vi "Get Log File Name And Path.vi"(6 "timeout (ms)":i32=-1, 8 "error in (no error)":errorcluster, 11 "FlexLogger_gRPCAPI in":refnum<class "FlexLogger_gRPC.lvclass">) -> (0 "error out":errorcluster, 2 "LogFileNamePath":T1, 3 "FlexLogger_gRPCAPI out":refnum<class "FlexLogger_gRPC.lvclass">)   [LabVIEW 2020, in "FlexLogger_gRPC.lvlib" / "FlexLogger_gRPC.lvclass"]
uses:
  FlexLogger_gRPC.lvclass
  Controls/FlexLogger File Name and Path.ctl
  FlexLogger_client/RPC Messages/flexlogger_GetLogFileBasePathRequest.ctl
  FlexLogger_client/RPC Messages/flexlogger_ElementIdentifier.ctl
  FlexLogger_gRPC.lvclass/FlexLogger_gRPC.ctl
  FlexLogger_client/FlexLogger_client.lvlib
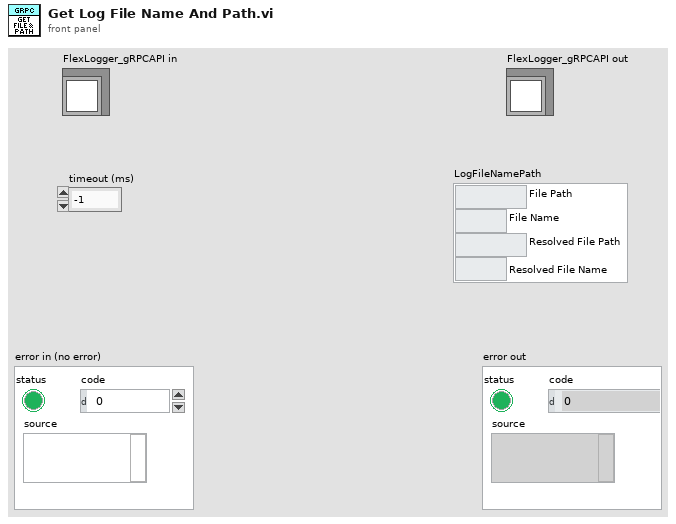
[diagram p1: front panel]
types:
  T1 = typedef "FlexLogger_gRPC.lvlib/FlexLogger_gRPC.lvclass/FlexLogger File Name and Path.ctl" = cluster{"File Path":string, "File Name":string, "Resolved File Path":string, "Resolved File Name":string}
  T2 = typedef "FlexLogger_client.lvlib/flexlogger_GetLogFileBasePathRequest.ctl" = cluster{"document_identifier":T3}
  T3 = typedef "FlexLogger_client.lvlib/flexlogger_ElementIdentifier.ctl" = cluster{"project_id":string, "file_name":string, "element_id":string, "subpart_id":string}
  T4 = typedef "grpc-lvsupport-release.lvlib/grpcId.ctl" = u64
  T5 = typedef "FlexLogger_client.lvlib/flexlogger_GetLogFileBasePathResponse.ctl" = cluster{"log_file_base_path":string}
  T6 = typedef "FlexLogger_client.lvlib/flexlogger_GetLogFileNameResponse.ctl" = cluster{"log_file_name":string}
  T7 = typedef "FlexLogger_client.lvlib/flexlogger_GetResolvedLogFileBasePathResponse.ctl" = cluster{"resolved_log_file_base_path":string}
  T8 = typedef "FlexLogger_client.lvlib/flexlogger_GetResolvedLogFileNameResponse.ctl" = cluster{"resolved_log_file_name":string}
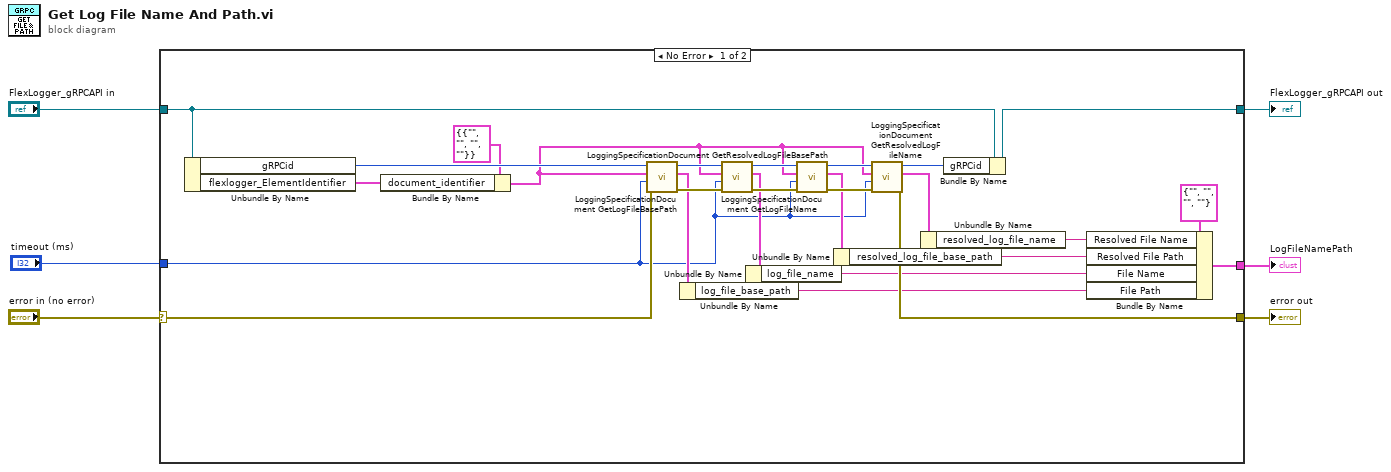
[diagram p0: block diagram]
diagram:
  n1 = case shown="No Error" "error in (no error)" {
    selector: "error in (no error)" -> [w8 w33]
    tunnel: "FlexLogger_gRPCAPI in" -> [w32 w34]
    tunnel: [w31 w34] -> w6
    tunnel: [w23 w33] -> w4
    tunnel: [w13 _] -> w2
    tunnel: "timeout (ms)" -> [w7 _]
    frame No Error {
      n2 = Unbundle By Name(w32) -> ("gRPCid"=w12:T4, "flexlogger_ElementIdentifier"=w10:T3)
      n3 = Bundle By Name(cluster=T2 {"document_identifier"={"project_id"="", "file_name"="", "element_id"="", "subpart_id"=""}} ("Request Data"), "document_identifier"=w10) -> (w9:T2)
      n4 = call "LoggingSpecificationDocument GetLogFileBasePath.vi"("error in"=w8, "timeout (ms)"=w7, "Request Data"=w9, "gRPC ID"=w12) -> ("error out"=w26:errorcluster, "Response Data"=w21:T5, "gRPC ID out"=w30:T4)  [unwired: 5 in]
      n5 = Unbundle By Name(w21) -> ("log_file_base_path"=w20:string)
      n6 = call "LoggingSpecificationDocument GetLogFileName.vi"("error in"=w26, "timeout (ms)"=w7, "Request Data"=w9, "gRPC ID"=w30) -> ("error out"=w25:errorcluster, "Response Data"=w19:T6, "gRPC ID out"=w29:T4)  [unwired: 5 in]
      n7 = Unbundle By Name(w19) -> ("log_file_name"=w18:string)
      n8 = call "LoggingSpecificationDocument GetResolvedLogFileBasePath.vi"("error in"=w25, "timeout (ms)"=w7, "Request Data"=w9, "gRPC ID"=w29) -> ("error out"=w24:errorcluster, "Response Data"=w17:T7, "gRPC ID out"=w28:T4)  [unwired: 5 in]
      n9 = Unbundle By Name(w17) -> ("resolved_log_file_base_path"=w16:string)
      n10 = call "LoggingSpecificationDocument GetResolvedLogFileName.vi"("error in"=w24, "timeout (ms)"=w7, "Request Data"=w9, "gRPC ID"=w28) -> ("error out"=w23:errorcluster, "Response Data"=w15:T8, "gRPC ID out"=w27:T4)  [unwired: 5 in]
      n11 = Unbundle By Name(w15) -> ("resolved_log_file_name"=w14:string)
      n12 = Bundle By Name(cluster=w32, "gRPCid"=w27) -> (w31:refnum<class "FlexLogger_gRPC.lvclass">)
      n13 = Bundle By Name(cluster=T1 {"File Path"="", "File Name"="", "Resolved File Path"="", "Resolved File Name"=""} ("LogFileNamePath"), "Resolved File Name"=w14, "Resolved File Path"=w16, "File Name"=w18, "File Path"=w20) -> (w13:T1)
    }
    frame Error {
    }
  }
  "error out" <- w4
  "FlexLogger_gRPCAPI out" <- w6
  "LogFileNamePath" <- w2
